vi "IMAQ FPGA Camera Link Data to Pixels 8 Tap 8-Bit.vi"(1 "Camera Link Data":T1) -> (0 "Pixels":u8[](array[numeric]))   [LabVIEW 2017]
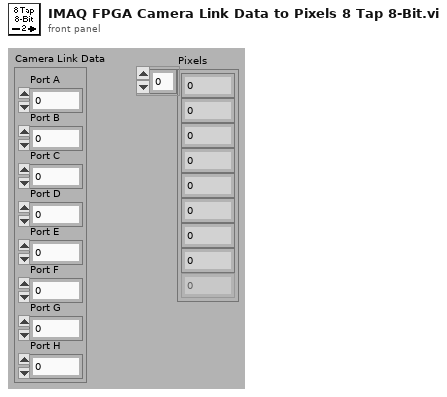
[diagram p1: front panel]
types:
  T1 = cluster{"Port A":u8, "Port B":u8, "Port C":u8, "Port D":u8, "Port E":u8, "Port F":u8, "Port G":u8, "Port H":u8}
  T2 = cluster{"Pixel 0":u8, "Pixel 1":u8, "Pixel 2":u8, "Pixel 3":u8, "Pixel 4":u8, "Pixel 5":u8, "Pixel 6":u8, "Pixel 7":u8}
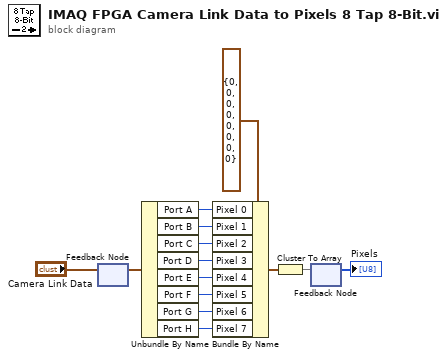
[diagram p0: block diagram]
diagram:
  n1 = feedback-in #1("Camera Link Data") -> ()
  n2 = feedback #1() -> (w11:T1)  [unwired: 1 in]
  n3 = Unbundle By Name(w11) -> ("Port A"=w10:u8, "Port B"=w9:u8, "Port C"=w8:u8, "Port D"=w7:u8, "Port E"=w6:u8, "Port F"=w5:u8, "Port G"=w4:u8, "Port H"=w3:u8)
  n4 = Bundle By Name(cluster=T2 {"Pixel 0"=0, "Pixel 1"=0, "Pixel 2"=0, "Pixel 3"=0, "Pixel 4"=0, "Pixel 5"=0, "Pixel 6"=0, "Pixel 7"=0} ("PixelData"), "Pixel 0"=w10, "Pixel 1"=w9, "Pixel 2"=w8, "Pixel 3"=w7, "Pixel 4"=w6, "Pixel 5"=w5, "Pixel 6"=w4, "Pixel 7"=w3) -> (w13:T2)
  n5 = Cluster To Array(cluster=w13) -> (array=w2:u8[])
  n6 = feedback #2() -> (→"Pixels":u8[])  [unwired: 1 in]
  n7 = feedback-in #2(w2) -> ()
